vi "COD质控流程 (子VI).vi"(10 "CODMn量程切换":enum32{"H", "L", "AUTO"}(ring)=enum."AUTO", 11 "COD":bool) -> (2 "CODMn中断报警":bool, 3 "布尔":bool)   [LabVIEW 2016, in "质控单元.lvlib"]
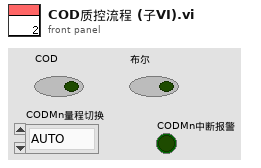
[diagram p1: front panel]
types:
  T1 = enum16{"待机", "启动水样测量", "水样测量中", "启动加标", "启动加标回收", "加标回收测量中", "结束"}
  T2 = cluster{"测量模式":enum16{"水样测量", "标样核查", "零点核查", "跨度核查", "空白测试", "加标回收", "平行样", "校零", "校标"}}
  T3 = enum16{"空闲", "水样测试", "标样核查", "零点核查", "跨度核查", "空白测试", "平行样测试", "质控样", "空白校准", "标样校准", "加标回收"}
  T4 = enum16{"空闲", "水样测试", "标样核查", "零点核查", "跨度核查", "空白测试", "平行样测试", "加标回收", "空白校准", "标样校准", "初始化（清洗）"}
  T5 = cluster{"量程":dbl, "检出限":dbl, "加标前水样浓度":dbl, "加标后水样浓度":dbl, "加标水杯定容体积":dbl, "加标母液浓度":dbl, "加标体积":dbl, "加标回收率":dbl}
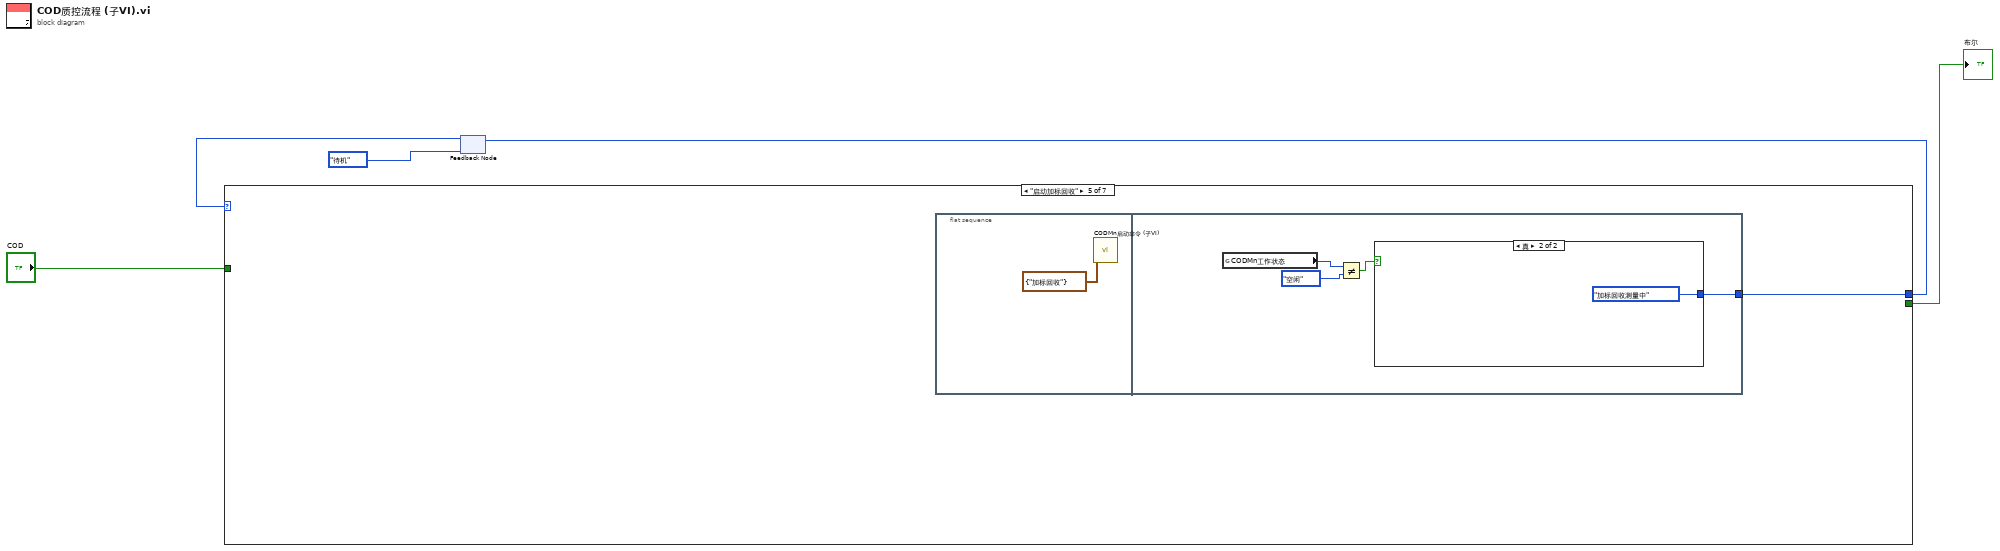
[diagram p0: block diagram]
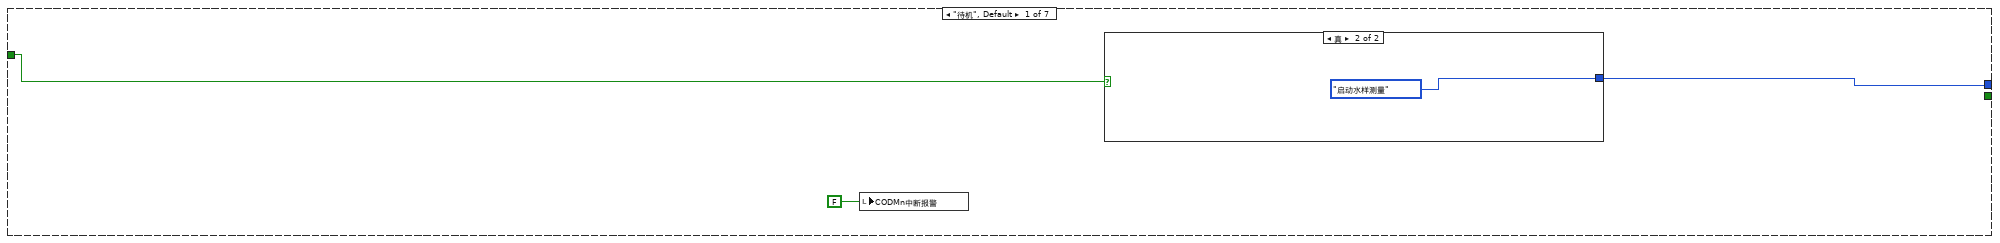
[diagram p2: hidden frame]
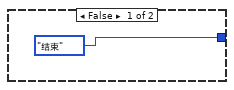
[diagram p3: hidden frame]
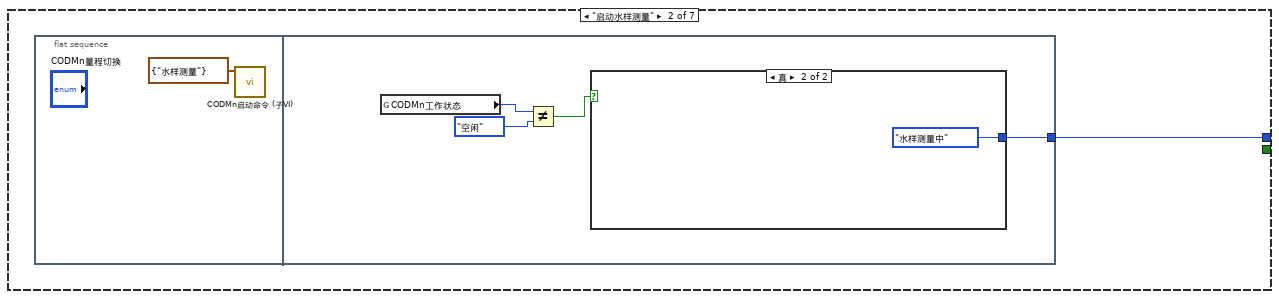
[diagram p4: hidden frame]
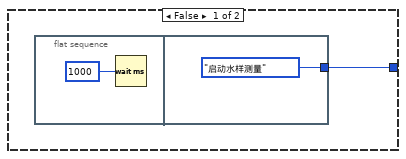
[diagram p5: hidden frame]
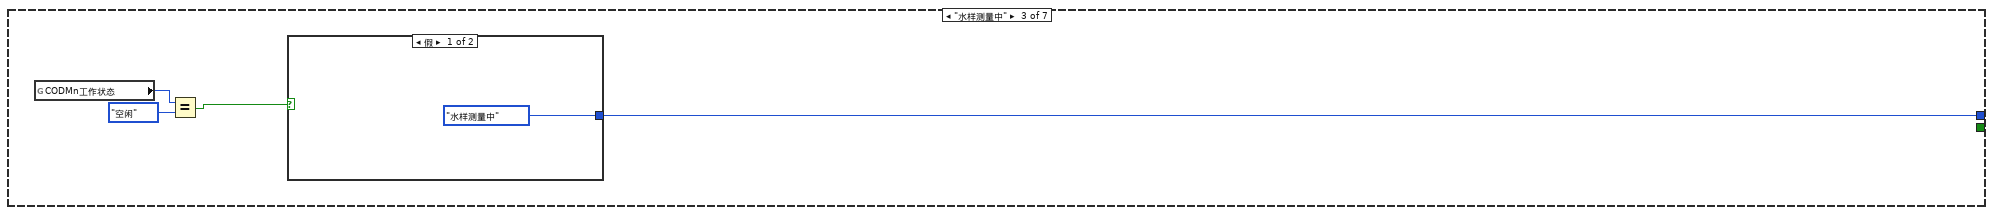
[diagram p6: hidden frame]
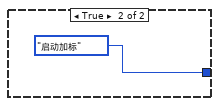
[diagram p7: hidden frame]
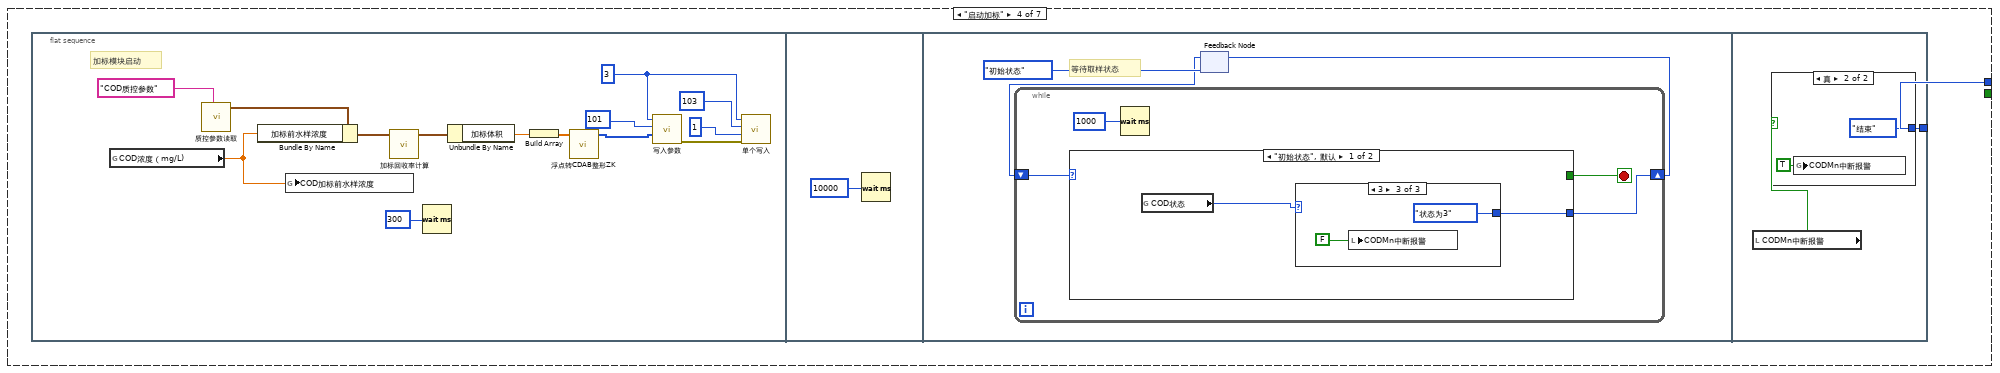
[diagram p8: hidden frame]
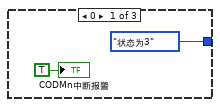
[diagram p9: hidden frame]
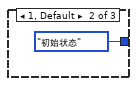
[diagram p10: hidden frame]
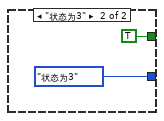
[diagram p11: hidden frame]
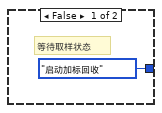
[diagram p12: hidden frame]
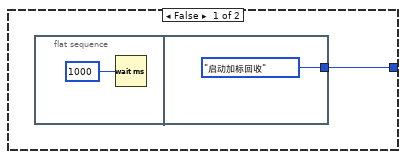
[diagram p13: hidden frame]
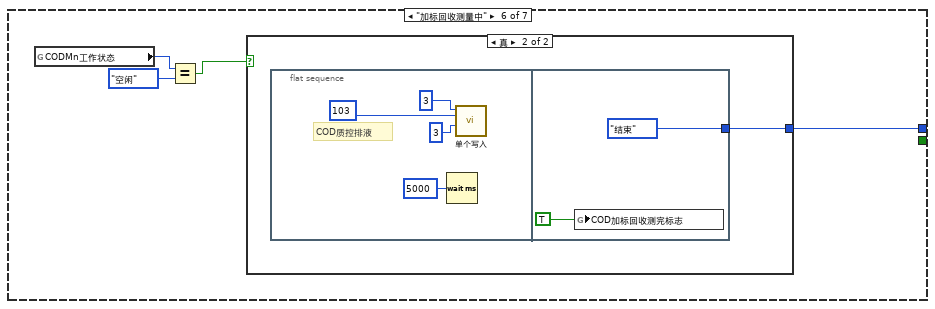
[diagram p14: hidden frame]
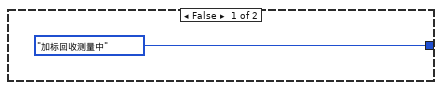
[diagram p15: hidden frame]
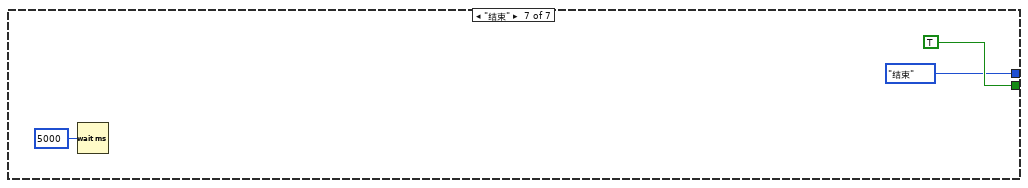
[diagram p16: hidden frame]
diagram:
  n1 = feedback #1(T1."待机") -> (w3:T1)
  n2 = case shown="\"启动加标回收\"" w3 {
    tunnel: [w8 w11 w24 w27 w64 w77 T1."结束"] -> w4
    tunnel: [_ _ _ _ _ _ TRUE] -> w2
    tunnel: "COD" -> [w7 _ _ _ _ _ _]
    frame "待机", Default {
      n3 = local write "CODMn中断报警"(FALSE ("CODMn中断报警")) -> ()
      n4 = case shown="真" w7 {
        tunnel: [T1."结束" T1."启动水样测量"] -> w8
        frame False {
        }
        frame True {
        }
      }
    }
    frame "启动水样测量" {
      n5 = flat-sequence {
        tunnel: [w16] -> w11
        frame #0 {
          n6 = call "CODMn启动命令 (子VI).vi"("启动测量模式"=T2 {"测量模式"=enum."水样测量"}) -> ()  [unwired: 10 in, 1 out]
        }
        frame #1 {
          n7 = global read "与CODMn交互全局.vi" "CODMn工作状态"() -> (w15:T4)
          n8 = Not Equal?(x=w15, y=T3."空闲") -> (x != y?=w13:bool)
          n9 = case shown="真" w13 {
            tunnel: [w17 T1."水样测量中"] -> w16
            frame False {
              n10 = flat-sequence {
                tunnel: [T1."启动水样测量"] -> w17
                frame #0 {
                  n11 = Wait (ms)(milliseconds to wait=u32 1000 ("等待时间（毫秒）")) -> ()  [unwired: 1 out]
                }
                frame #1 {
                }
              }
            }
            frame True {
            }
          }
        }
      }
    }
    frame "水样测量中" {
      n12 = global read "与CODMn交互全局.vi" "CODMn工作状态"() -> (w23:T4)
      n13 = Equal?(x=w23, y=T3."空闲") -> (x = y?=w21:bool)
      n14 = case shown="假" w21 {
        tunnel: [T1."水样测量中" T1."启动加标"] -> w24
        frame False {
        }
        frame True {
        }
      }
    }
    frame "启动加标" {
      n15 = flat-sequence {
        tunnel: [w60] -> w27
        frame #0 {
          w29 = u16 3 ("value")
          # "加标模块启动"
          n16 = global read "与CODMn交互全局.vi" "COD浓度（mg/L)"() -> (w30:dbl)
          n17 = call "质控参数读取.vi"("section"="COD质控参数") -> ("参数"=w39:T5)  [unwired: 9 in, 1 out]
          n18 = Bundle By Name(cluster=w39, "加标前水样浓度"=w30) -> (w40:T5)
          n19 = global write "水样浓度全局.vi" "COD加标前水样浓度"(w30) -> ()
          n20 = call "加标回收率计算.vi"("参数"=w40) -> ("参数 out"=w38:T5)  [unwired: 10 in]
          n21 = Wait (ms)(milliseconds to wait=u32 300 ("等待时间（毫秒）")) -> ()  [unwired: 1 out]
          n22 = Unbundle By Name(w38) -> ("加标体积"=w31:dbl)
          n23 = Build Array(w31) -> (w37:dbl[])
          n24 = call "浮点转CDAB整形ZK.vi"("浮点数"=w37) -> ("CDAB整形输出"=w32:u16[])  [unwired: 10 in]
          n25 = call "写入参数.vi"("values"=w32, "starting address"=u16 101, "Slave ID"=w29) -> ("error out"=w36:errorcluster)  [unwired: 8 in]
          n26 = call "单个写入.vi"("Error in"=w36, "value"=u16 1, "address"=u16 103, "Slave ID"=w29) -> ()  [unwired: 7 in, 1 out]
        }
        frame #1 {
          n27 = Wait (ms)(milliseconds to wait=u32 10000 ("等待时间（毫秒）")) -> ()  [unwired: 1 out]
        }
        frame #2 {
          # "等待取样状态"
          n28 = feedback #2(enum16{"初始状态", "状态为3"}."初始状态") -> (w44:enum16{"初始状态", "状态为3"})
          n29 = while {
            shift-right: [w48] -> w43
            shift-left: w44 -> [w49]
            stop <- w47 stop-if-true
            n30 = case shown="\"初始状态\", 默认" w49 {
              tunnel: [w51 enum16{"初始状态", "状态为3"}."状态为3"] -> w48
              tunnel: [_ TRUE] -> w47
              frame "初始状态", Default {
                n31 = global read "加标回收状态全局变量.vi" "COD状态"() -> (w50:u16)
                n32 = case shown="3" w50 {
                  tunnel: [enum16{"初始状态", "状态为3"}."状态为3" enum16{"初始状态", "状态为3"}."初始状态" enum16{"初始状态", "状态为3"}."状态为3"] -> w51
                  frame 0 {
                    "CODMn中断报警" <- TRUE ("CODMn中断报警")
                  }
                  frame 1, Default {
                  }
                  frame 3 {
                    n33 = local write "CODMn中断报警"(FALSE ("CODMn中断报警")) -> ()
                  }
                }
              }
              frame "状态为3" {
              }
            }
            n34 = Wait (ms)(milliseconds to wait=u32 1000 ("等待时间（毫秒）")) -> ()  [unwired: 1 out]
          }
          n35 = feedback-in #2(w43) -> ()
        }
        frame #3 {
          n36 = local read "CODMn中断报警"() -> (w59:bool)
          n37 = case shown="真" w59 {
            tunnel: [T1."启动加标回收" T1."结束"] -> w60
            frame False {
              # "等待取样状态"
            }
            frame True {
              n38 = global write "质控中断报警全局.vi" "CODMn中断报警"(TRUE ("CODMn中断报警")) -> ()
            }
          }
        }
      }
    }
    frame "启动加标回收" {
      n39 = flat-sequence {
        tunnel: [w69] -> w64
        frame #0 {
          n40 = call "CODMn启动命令 (子VI).vi"("启动测量模式"=T2 {"测量模式"=enum."加标回收"}) -> ()  [unwired: 10 in, 1 out]
        }
        frame #1 {
          n41 = global read "与CODMn交互全局.vi" "CODMn工作状态"() -> (w68:T4)
          n42 = Not Equal?(x=w68, y=T3."空闲") -> (x != y?=w66:bool)
          n43 = case shown="真" w66 {
            tunnel: [w70 T1."加标回收测量中"] -> w69
            frame False {
              n44 = flat-sequence {
                tunnel: [T1."启动加标回收"] -> w70
                frame #0 {
                  n45 = Wait (ms)(milliseconds to wait=u32 1000 ("等待时间（毫秒）")) -> ()  [unwired: 1 out]
                }
                frame #1 {
                }
              }
            }
            frame True {
            }
          }
        }
      }
    }
    frame "加标回收测量中" {
      n46 = global read "与CODMn交互全局.vi" "CODMn工作状态"() -> (w76:T4)
      n47 = Equal?(x=w76, y=T3."空闲") -> (x = y?=w74:bool)
      n48 = case shown="真" w74 {
        tunnel: [T1."加标回收测量中" w79] -> w77
        frame False {
        }
        frame True {
          n49 = flat-sequence {
            tunnel: [T1."结束"] -> w79
            frame #0 {
              # "COD质控排液"
              n50 = Wait (ms)(milliseconds to wait=u32 5000 ("等待时间（毫秒）")) -> ()  [unwired: 1 out]
              n51 = call "单个写入.vi"("value"=u16 3, "address"=u16 103, "Slave ID"=u8 3) -> ()  [unwired: 8 in, 1 out]
            }
            frame #1 {
              n52 = global write "质控测完标志全局 1.vi" "COD加标回收测完标志"(TRUE ("COD加标回收测完标志")) -> ()
            }
          }
        }
      }
    }
    frame "结束" {
      n53 = Wait (ms)(milliseconds to wait=u32 5000 ("等待时间（毫秒）")) -> ()  [unwired: 1 out]
    }
  }
  "布尔" <- w2
  n54 = feedback-in #1(w4) -> ()
